vi "RP block write.vi"(8 "Error In":errorcluster, 10 "Data":i16[](array[numeric]), 11 "connection ID":refnum<k5>) -> (0 "Error Out":errorcluster, 3 "connection ID out":refnum<k5>)   [LabVIEW 2024]
uses:
  RP Command.ctl
  RP Write Command TCP.vi
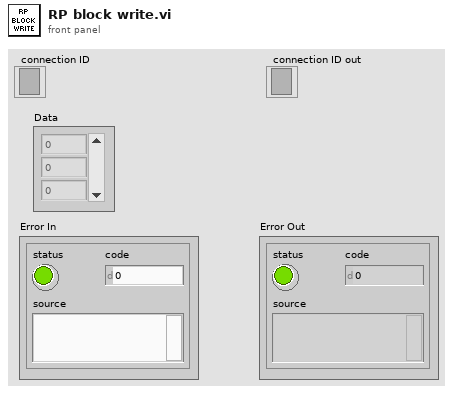
[diagram p1: front panel]
types:
  T1 = typedef "RP Command.ctl" = enum16{"Reset", "Read IDN", "Stop server", "Get status", "Get temperature", "Connect client", "Arm", "Software trigger", "Get whole buffer", "Get chunk", "System call", "Get config", "Set config", "Recieve data", "Recieve Calibartion", "Transmit data"}
  T2 = enum16{"big-endian, network order", "native, host order", "little-endian"}
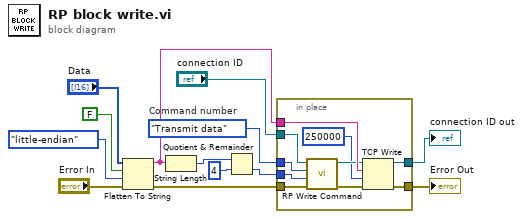
[diagram p0: block diagram]
diagram:
  w4 = RP_Command."Transmit data"  # Command number
  n1 = Flatten To String(anything="Data", prepend array or string size? (T)=FALSE, byte order (0:big-endian, network order)=T2."little-endian", error in (no error)="Error In") -> (data string=w9:string, error out=w5:errorcluster)  [unwired: 1 out]
  n2 = String Length(string=w9) -> (length=w2:i32)
  n3 = Quotient & Remainder(x=w2, y=4) -> (floor(x/y)=w3:i32)  [unwired: 1 out]
  n4 = in-place {
    in-place-border: "connection ID" -> [w23]
    in-place-border: w9 -> [w22]
    in-place-border: [w20] -> w8
    in-place-border: [w19] -> w7
    in-place-border: w5 -> [w18]
    in-place-border: w4 -> [w16]
    in-place-border: w3 -> [w15]
    n5 = call-poly "RP Write Command.vi"("Error In"=w18, "Command payload"=w15, "Command number"=w16, "connection ID"=w23) -> ("Error Out"=w17:errorcluster, "connection ID out"=w21:refnum<k5>)  [unwired: 4 in, 2 out]
    n6 = TCP Write(connection ID=w21, data in=w22, error in (no error)=w17, 9:250000 ("timeout ms (25000)")) -> (connection ID out=w19:refnum<k5>, error out=w20:errorcluster)  [unwired: 1 out]
  }
  "connection ID out" <- w7
  "Error Out" <- w8
